vi "from string array.vi"(8 "error in (no error)":errorcluster, 9 "String Array":string[][](array[string]), 10 "version":string, 11 "module configuration in":refnum<class "Modbus Module configuration.lvclass">) -> (0 "error out":errorcluster, 3 "module configuration out":refnum<class "Modbus Module configuration.lvclass">)   [LabVIEW 2015, in "Modbus Module configuration.lvclass"]
uses:
  Modbus Module configuration.lvclass
  module channel/Modbus Module Channel.lvclass
  <vilib>/NI/Tag Bus/tag/Data Type.ctl
  editor node/permissions.ctl
  <vilib>/NI/Tag Bus/tag/tag descriptor.lvclass/tag descriptor.ctl
  <vilib>/NI/Tag Bus Module Framework/channel/TBM channel.lvclass/TBM channel.ctl
  Modbus Module configuration.lvclass/Modbus Module configuration.ctl
  <vilib>/NI/Tag Bus/tag/tag descriptor.lvclass
  editor node/Modbus Module editor node.lvclass
  <vilib>/NI/Tag Bus Module Framework/channel/TBM channel.lvclass
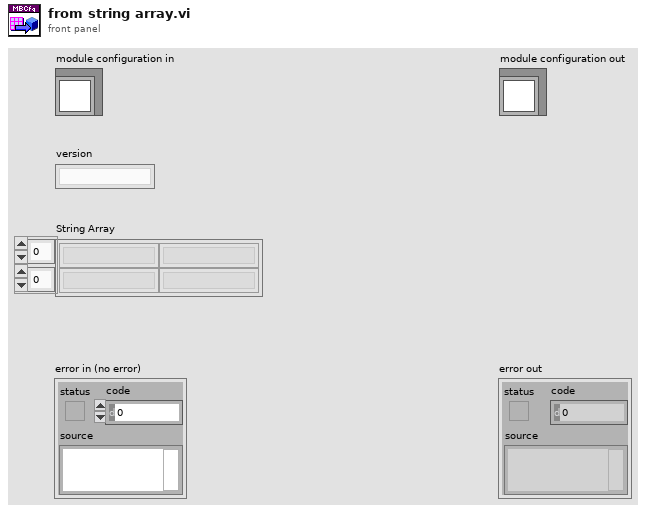
[diagram p1: front panel]
types:
  T1 = typedef "Modbus Module editor node.lvclass/permissions.ctl" = enum32{"Read from MB", "Write to MB"}
  T2 = typedef "tag bus.lvlib/tag descriptor.lvclass/Data Type.ctl" = enum16{"Double", "Single", "I64", "I32", "I16", "I8", "U64", "U32", "U16", "U8", "Boolean", "String", "Array of Double", "Array of Single", "Array of I64", "Array of I32", "Array of I16", "Array of I8", "Array of U64", "Array of U32", "Array of U16", "Array of U8", "Array of Boolean", "Array of String"}
  T3 = typedef "TBM channel.lvclass/channel classification.ctl" = enum16{"input data", "output data", "processing parameter", "processing result"}
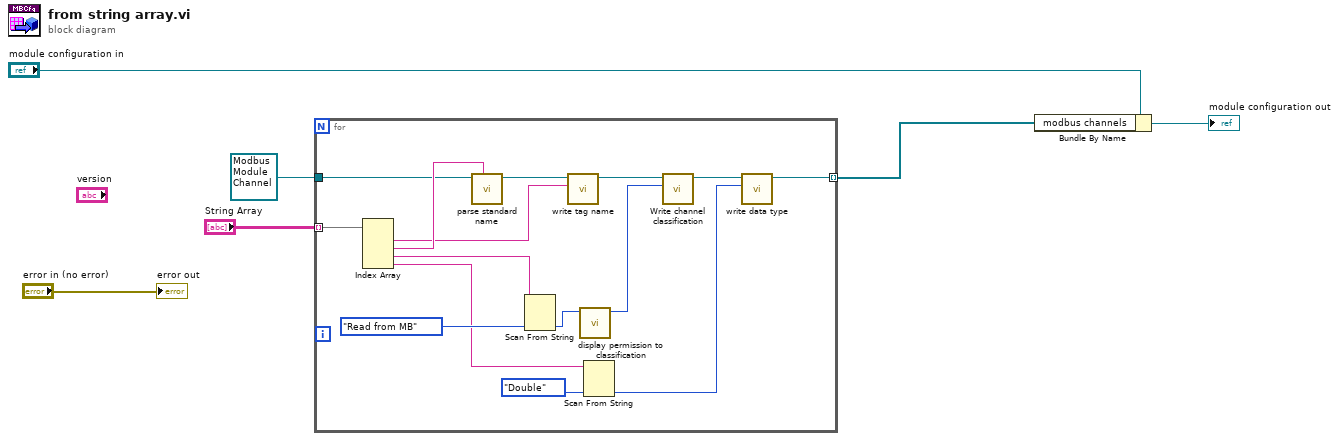
[diagram p0: block diagram]
diagram:
  n1 = for {
    tunnel: "String Array" -> [w21] mode=indexing
    tunnel: refnum<class "Modbus Module Channel.lvclass"> refnum ("Modbus Module Channel in") -> [w14]
    tunnel: [w8] -> w2 mode=indexing
    n2 = Index Array(array=w21) -> (element #1=w12:string, element #2=w15:string, element #3=w19:string, element #4=w16:string)  [unwired: 4 in]
    n3 = call "parse standard name.vi"("standard name"=w15, "Modbus Module Channel in"=w14) -> ("Modbus Module Channel out"=w13:refnum<class "Modbus Module Channel.lvclass">)  [unwired: 8 in, 1 out]
    n4 = Scan From String(input string=w19, default 1=permissions."Read from MB" ("permissions")) -> (output 1=w17:T1)  [unwired: 3 in, 3 out]
    n5 = call <vilib>:"write tag name.vi"("name"=w12, "system tag in"=w13) -> ("system tag out"=w11:refnum<class "Modbus Module Channel.lvclass">)  [unwired: 8 in, 1 out]
    n6 = call "display permission to classification.vi"("display permissions"=w17) -> ("channel classification"=w10:T3)  [unwired: 10 in]
    n7 = Scan From String(input string=w16, default 1=Data_Type."Double" ("data type")) -> (output 1=w7:T2)  [unwired: 3 in, 3 out]
    n8 = call <vilib>:"Write channel classification.vi"("channel classification"=w10, "channel in"=w11) -> ("channel out"=w9:refnum<class "Modbus Module Channel.lvclass">)  [unwired: 8 in, 1 out]
    n9 = call <vilib>:"write data type.vi"("data type"=w7, "system tag in"=w9) -> ("system tag out"=w8:refnum<class "Modbus Module Channel.lvclass">)  [unwired: 8 in, 1 out]
  }
  n10 = Bundle By Name(cluster="module configuration in", "modbus channels"=w2) -> (→"module configuration out":refnum<class "Modbus Module configuration.lvclass">)
  "error out" <- "error in (no error)"
